vi "SaveString.vi"(2 "input string":string="C:\\SlowCtrl\\data\\", 3 "filename":string="_pres.txt", 5 "directory name":string="C:\\SlowCtrl\\data\\") -> ()   [LabVIEW 2017]
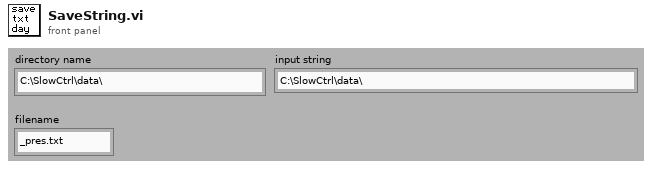
[diagram p1: front panel]
types:
  T1 = enum16{"open", "replace", "create", "open or create", "replace or create", "replace or create with confirmation"}
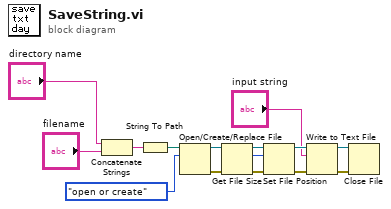
[diagram p0: block diagram]
diagram:
  n1 = Concatenate Strings("directory name", "filename") -> (w13:string)
  n2 = String To Path(string=w13) -> (path=w2:path)
  n3 = Open/Create/Replace File(file path (use dialog)=w2, operation (0:open)=T1."open or create" ("操作 (0:開く)")) -> (refnum out=w11:refnum<file>, error out=w6:errorcluster)  [unwired: 4 in, 1 out]
  n4 = Get File Size(file=w11, error in=w6) -> (refnum out=w7:refnum<file>, size (in bytes)=w12:i64, 0:w8:errorcluster)
  n5 = Set File Position(offset (in bytes) (0)=w12, refnum=w7, error in=w8) -> (refnum out=w9:refnum<file>, error out=w10:errorcluster)  [unwired: 1 in]
  n6 = Write to Text File(file (use dialog)=w9, text="input string", error in=w10) -> (refnum out=w5:refnum<file>, error out=w4:errorcluster)  [unwired: 1 in, 1 out]
  n7 = Close File(refnum=w5, error in=w4) -> ()  [unwired: 2 out]
